vi "Loop Stack Recursion.vi"() -> ()   [LabVIEW 2011]
uses:
  <userlib>/_OpenG.lib/lvdata/lvdata.llb/Type Descriptor Enumeration__ogtk.ctl
panel:
  in  "outer cluster":T1={"str1"="hello", "str2"="world", "inner cluster"={"str3"="foo", "str4"="bar"}, "inner array"=[{"str5"="foo", "str6"="bar", "Numeric"=0.0}]}
  out "element":variant
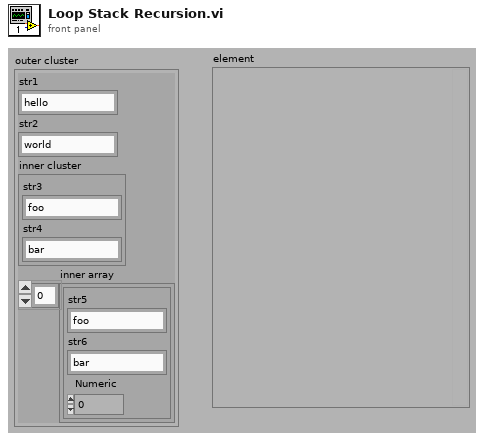
[diagram p1: front panel]
types:
  T1 = cluster{"str1":string, "str2":string, "inner cluster":cluster{"str3":string, "str4":string}, "inner array":cluster{"str5":string, "str6":string, "Numeric":dbl}[]}
  T2 = typedef "Type Descriptor Enumeration__ogtk.ctl" = enum8{"<Null>", "I8", "I16", "I32", "I64", "U8", "U16", "U32", "U64", "SGL", "DBL", "EXT", "CSG", "CDB", "CXT", "0x0F", "0x10", "0x11", "0x12", "0x13", "0x14", "Enum U8", "Enum U16", "Enum U32", "Enum U64", "SGL PQ", "DBL PQ", "EXT PQ", "CSG PQ", "CDB PQ", "CXT PQ", "0x1F", "0x20", "Boolean", "0x22", "0x23", "0x24", "0x25", "0x26", "0x27", "0x28", "0x29", "0x2A", "0x2B", "0x2C", "0x2D", "0x2E", "0x2F", "String", "0x31", "Path", "Pict", "0x34", "0x35", "0x36", "DAQ", "0x38", "0x39", "0x3A", "0x3B", "0x3C", "0x3D", "0x3E", "0x3F", "Array", "0x41", "0x42", "0x43", "0x44", "0x45", "0x46", "0x47", "0x48", "0x49", "0x4A", "0x4B", "0x4C", "0x4D", "0x4E", "0x4F", "Cluster", "0x51", "0x52", "Variant", "Waveform", "0x55", "0x56", "0x57", "0x58", "0x59", "0x5A", "0x5B", "0x5C", "0x5D", "0x5E", "0x5F", "0x60", "0x61", "0x62", "0x63", "0x64", "0x65", "0x66", "0x67", "0x68", "0x69", "0x6A", "0x6B", "0x6C", "0x6D", "0x6E", "0x6F", "Refnum"}
  T3 = cluster{"Data Name":string, "Type Descriptor Enumeration":T2, i32}
  T4 = cluster{"Data Name":string, "Type Descriptor Enumeration":T2, "level":i32}[]
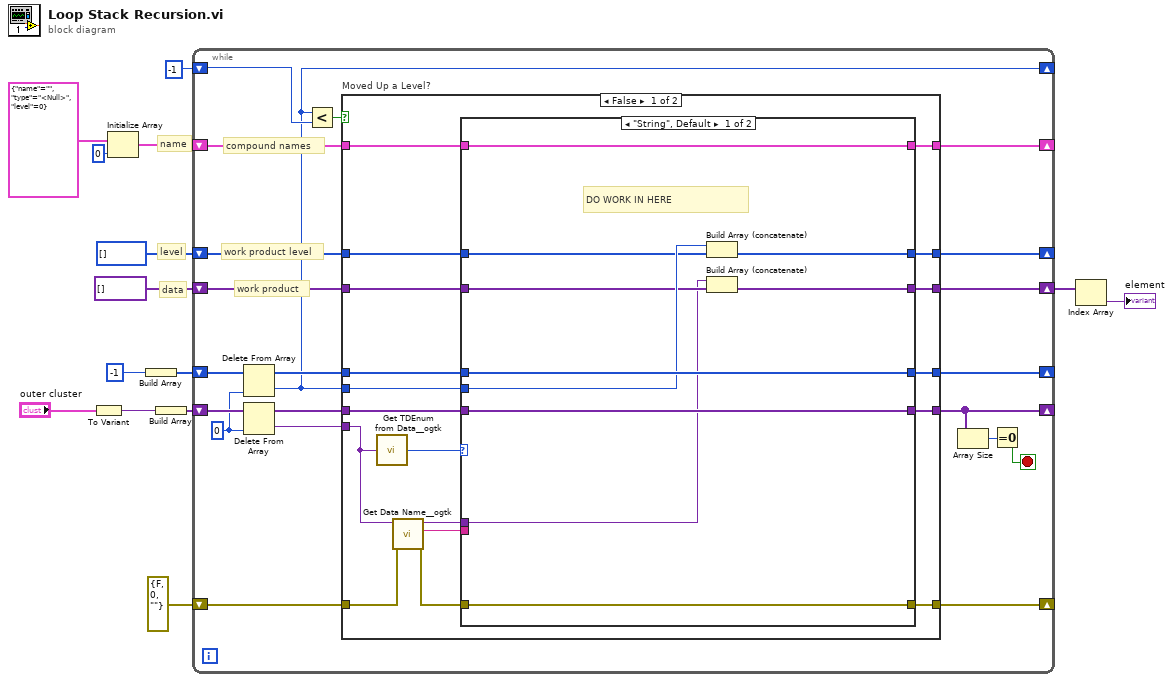
[diagram p0: block diagram]
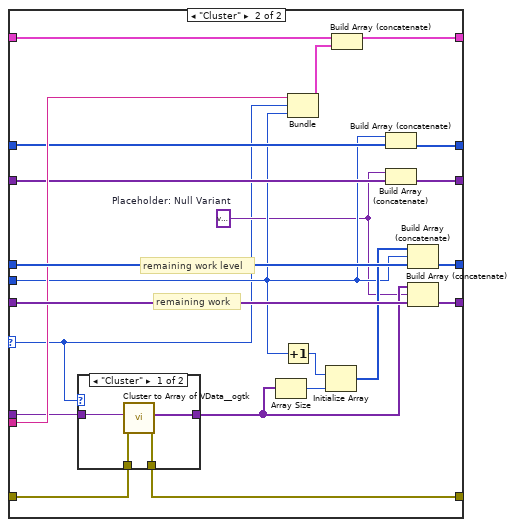
[diagram p2: hidden frame]
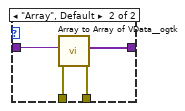
[diagram p3: hidden frame]
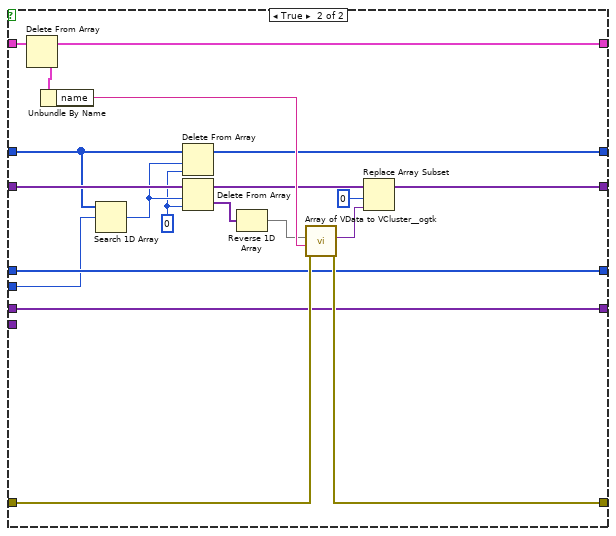
[diagram p4: hidden frame]
diagram:
  # "name"
  # "level"
  # "data"
  n1 = To Variant(anything="outer cluster") -> (Variant=w12:variant)
  n2 = Initialize Array(cluster{"name":string, "type":T2, "level":i32} {"name"="", "type"=enum."<Null>", "level"=0}, 0 ("dimension size")) -> (w3:cluster{"name":string, "type":T2, "level":i32}[])
  n3 = Build Array(-1) -> (w8:i32[])
  n4 = Build Array(w12) -> (w14:variant[])
  n5 = while {
    shift-right: [w21] -> _
    shift-left: w14 -> [w35]
    shift-right: [w22] -> _
    shift-left: errorcluster {"status"=FALSE, "code"=0, "source"=""} ("error out") -> [w25]
    shift-right: [w18] -> w2
    shift-left: variant[] [] ("appended array") -> [w26]
    shift-right: [w19] -> _
    shift-left: i32[] [] -> [w27]
    shift-right: [w20] -> _
    shift-left: w3 -> [w29]
    shift-right: [w16] -> _
    shift-left: w8 -> [w31]
    shift-right: [w15] -> _
    shift-left: -1 -> [w28]
    stop <- w33 stop-if-true
    w32 = 0 ("index")
    # "compound names"
    # "work product level"
    # "work product"
    n6 = Delete From Array(array=w31, index=w32) -> (deleted portion=w15:i32, array with subset deleted=w17:i32[])  [unwired: 1 in]
    n7 = Delete From Array(array=w35, index=w32) -> (deleted portion=w24:variant, array with subset deleted=w23:variant[])  [unwired: 1 in]
    n8 = Less?(x=w15, y=w28) -> (x < y?=w30:bool)
    n9 = case "Moved Up a Level?" shown="False" w30 {
      tunnel: w29 -> [w37 w113]
      tunnel: [w36 w112] -> w20
      tunnel: w27 -> [w39 w98]
      tunnel: w26 -> [w41 w110]
      tunnel: [w40 w108] -> w18
      tunnel: [w38 w97] -> w19
      tunnel: [w46 w105] -> w22
      tunnel: w25 -> [w47 w104]
      tunnel: w24 -> [w49 _]
      tunnel: w23 -> [w48 w103]
      tunnel: [w45 w103] -> w21
      tunnel: w17 -> [w44 w102]
      tunnel: [w43 w102] -> w16
      tunnel: w15 -> [w42 w94]
      frame False {
        n10 = call <userlib>:"Get TDEnum from Data__ogtk.vi"("Data"=w49) -> ("Type Descriptor Enumeration"=w53:T2)  [unwired: 4 in]
        n11 = call <userlib>:"Get Data Name__ogtk.vi"("error in (no error)"=w47, "Data"=w49) -> ("error out"=w50:errorcluster, "Data Name"=w51:string, "Data dup"=w52:variant)  [unwired: 7 in]
        n12 = case shown="\"String\", Default" w53 {
          selector: w53 -> [_ w64]
          tunnel: w50 -> [w63 w85]
          tunnel: [w63 w84] -> w46
          tunnel: w52 -> [w54 w75]
          tunnel: w48 -> [w60 w83]
          tunnel: [w60 w82] -> w45
          tunnel: w51 -> [_ w78]
          tunnel: w37 -> [w62 w77]
          tunnel: [w62 w81] -> w36
          tunnel: w41 -> [w56 w70]
          tunnel: [w61 w69] -> w40
          tunnel: w39 -> [w55 w67]
          tunnel: [w59 w68] -> w38
          tunnel: w44 -> [w58 w80]
          tunnel: w42 -> [w57 w66]
          tunnel: [w58 w79] -> w43
          frame "String", Default {
            # "DO WORK IN HERE"
            n13 = Build Array (concatenate)(w57, w55) -> (w59:i32[])
            n14 = Build Array (concatenate)(w54, w56) -> (w61:variant[])
          }
          frame "Cluster" {
            w65 = variant  # Placeholder: Null Variant
            # "remaining work level"
            # "remaining work"
            n15 = case shown="\"Cluster\"" w64 {
              tunnel: w85 -> [w89 w93]
              tunnel: [w88 w92] -> w84
              tunnel: w75 -> [w87 w91]
              tunnel: [w86 w90] -> w72
              frame "Cluster" {
                n16 = call <userlib>:"Cluster to Array of VData__ogtk.vi"("error in (no error)"=w89, "Cluster"=w87) -> ("error out"=w88:errorcluster, "Array of VData"=w86:variant[])  [unwired: 8 in]
              }
              frame "Array", Default {
                n17 = call <userlib>:"Array to Array of VData__ogtk.vi"("error in (no error)"=w93, "MultiD Array"=w91) -> ("error out"=w92:errorcluster, "1D Array of Variants"=w90:variant[])  [unwired: 8 in]
              }
            }
            n18 = Array Size(array=w72) -> (size(s)=w71:i32)
            n19 = Increment(x=w66) -> (x+1=w74:i32)
            n20 = Bundle("Data Name"=w78, "Type Descriptor Enumeration"=w64, w66) -> (w76:T3)  [unwired: 1 in]
            n21 = Initialize Array(w74, w71) -> (w73:i32[])
            n22 = Build Array (concatenate)(w77, w76) -> (w81:T4)
            n23 = Build Array (concatenate)(w66, w67) -> (w68:i32[])
            n24 = Build Array (concatenate)(w65, w70) -> (w69:variant[])
            n25 = Build Array (concatenate)(w73, w66, w80) -> (w79:i32[])
            n26 = Build Array (concatenate)(w72, w65, w83) -> (w82:variant[])
          }
        }
      }
      frame True {
        w95 = 0 ("index")
        n27 = Delete From Array(array=w113) -> (deleted portion=w111:cluster{"name":string, "type":T2, "level":i32}, array with subset deleted=w112:cluster{"name":string, "type":T2, "level":i32}[])  [unwired: 2 in]
        n28 = Unbundle By Name(w111) -> ("name"=w109:string)
        n29 = Search 1D Array(1D array=w98, element=w94) -> (index of element=w96:i32)  [unwired: 1 in]
        n30 = Delete From Array(array=w98, length=w96, index=w95) -> (array with subset deleted=w97:i32[])  [unwired: 1 out]
        n31 = Delete From Array(array=w110, length=w96, index=w95) -> (deleted portion=w101:variant[], array with subset deleted=w99:variant[])
        n32 = Reverse 1D Array(array=w101) -> (reversed array=w100:variant[])
        n33 = call <userlib>:"Array of VData to VCluster__ogtk.vi"("error in (no error)"=w104, "Cluster Name"=w109, "Array"=w100) -> ("error out"=w105:errorcluster, "VCluster"=w106:variant)  [unwired: 7 in]
        n34 = Replace Array Subset(array=w99, new element=w106, index=0) -> (w108:variant[])
      }
    }
    n35 = Array Size(array=w21) -> (size(s)=w34:i32)
    n36 = Equal To 0?(x=w34) -> (x = 0?=w33:bool)
  }
  n37 = Index Array(array=w2) -> (element=→"element":variant)  [unwired: 1 in]
